vi "parsecommandtest.vi"() -> ()   [LabVIEW 2019, in "Instrument.OxfordVRM.lvclass"]
uses:
  Instrument.OxfordVRM.lvclass
  Typedefs/Instrument.VRM.protectedCommands-enum.ctl
  Typedefs/Instrument.VRM.publicCommands-enum.ctl
panel:
  out "String":string
  in  "input string":string
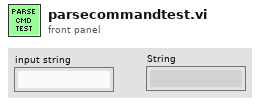
[diagram p1: front panel]
types:
  T1 = typedef "Instrument.OxfordVRM.lvclass/Instrument.VRM.protectedCommands-enum.ctl" = enum16{"Hold", "RampToSet", "RampToZero", "Clamp", "SetTarget", "GetStatus", "GetTarget", "GetField"}
  T2 = typedef "Instrument.OxfordVRM.lvclass/Instrument.VRM.publicCommands-enum.ctl" = enum16{"setMagnet", "setMagnetVector", "getMagnet", "getMagnetVector"}
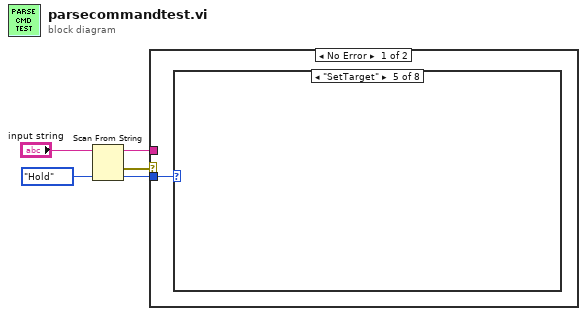
[diagram p0: block diagram]
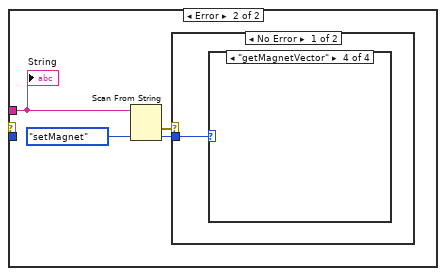
[diagram p9: hidden frame]
diagram:
  n1 = Scan From String(input string="input string", default 1=Instrument.VRM.protectedCommands-enum."Hold" ("protectedCommands")) -> (remaining string=w1:string, error out=w2:errorcluster, output 1=w3:T1)  [unwired: 3 in, 1 out]
  n2 = case shown="No Error" w2 {
    tunnel: w3 -> [w6 _]
    tunnel: w1 -> [_ w9]
    frame No Error {
      n3 = case shown="\"SetTarget\"" w6 {
        frame "Hold", Default {
        }
        frame "RampToSet" {
        }
        frame "RampToZero" {
        }
        frame "Clamp" {
        }
        frame "SetTarget" {
        }
        frame "GetStatus" {
        }
        frame "GetTarget" {
        }
        frame "GetField" {
        }
      }
    }
    frame Error {
      n4 = Scan From String(input string=w9, default 1=Instrument.VRM.publicCommands-enum."setMagnet" ("Commands")) -> (error out=w7:errorcluster, output 1=w8:T2)  [unwired: 3 in, 2 out]
      n5 = case shown="No Error" w7 {
        tunnel: w8 -> [w11 _]
        frame No Error {
          n6 = case shown="\"getMagnetVector\"" w11 {
            frame "setMagnet", Default {
            }
            frame "setMagnetVector" {
            }
            frame "getMagnet" {
            }
            frame "getMagnetVector" {
            }
          }
        }
        frame Error {
        }
      }
      "String" <- w9
    }
  }
